vi "DHE_ParseBinning.vi"(8 "error in":errorcluster, 10 "binning":string) -> (0 "error out":errorcluster, 2 "ybining":i32, 3 "xbining":i32)   [LabVIEW 2016]
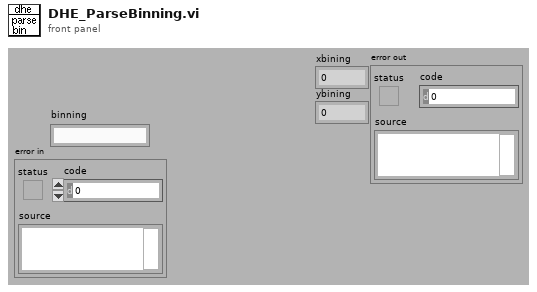
[diagram p1: front panel]
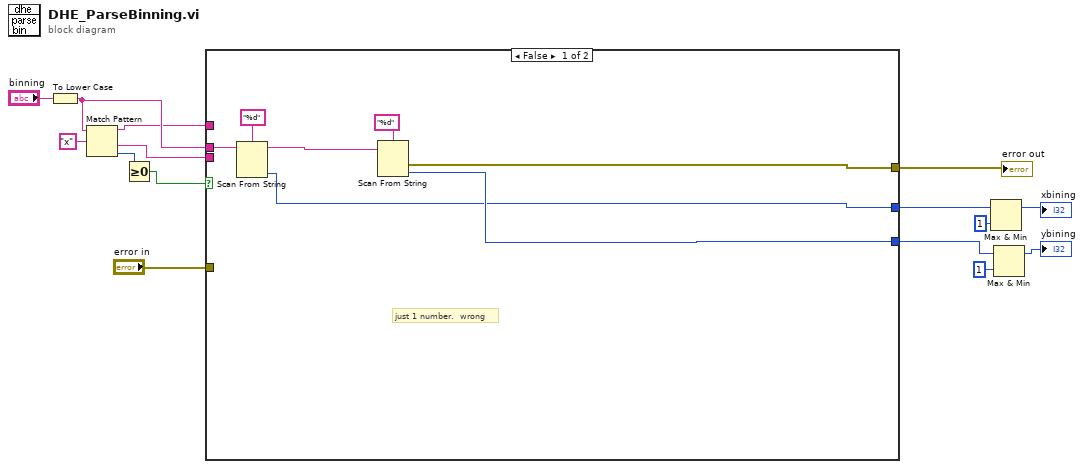
[diagram p0: block diagram]
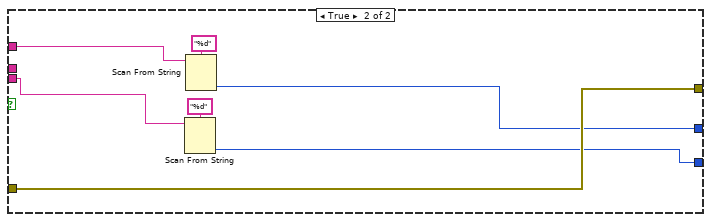
[diagram p2: hidden frame]
diagram:
  n1 = To Lower Case(string="binning") -> (all lower case string=w4:string)
  n2 = Match Pattern(string=w4, regular expression="x") -> (before substring=w2:string, after substring=w1:string, offset past match=w7:i32)  [unwired: 2 out]
  n3 = Greater Or Equal To 0?(x=w7) -> (x >= 0?=w3:bool)
  n4 = case shown="False" w3 {
    tunnel: [w20 w25] -> w15
    tunnel: "error in" -> [_ w25]
    tunnel: [w19 w23] -> w13
    tunnel: [w18 w24] -> w11
    tunnel: w4 -> [w17 _]
    tunnel: w2 -> [_ w27]
    tunnel: w1 -> [_ w26]
    frame False {
      # "just 1 number.  wrong"
      n5 = Scan From String(format string="%d", input string=w17) -> (remaining string=w21:string, output 1=w18:i32)  [unwired: 2 in, 3 out]
      n6 = Scan From String(format string="%d", input string=w21) -> (error out=w20:errorcluster, output 1=w19:i32)  [unwired: 2 in, 3 out]
    }
    frame True {
      n7 = Scan From String(format string="%d", input string=w26) -> (output 1=w23:i32)  [unwired: 2 in, 4 out]
      n8 = Scan From String(format string="%d", input string=w27) -> (output 1=w24:i32)  [unwired: 2 in, 4 out]
    }
  }
  "error out" <- w15
  n9 = Max & Min(x=w11, y=1) -> (max(x,y)=→"xbining":i32)  [unwired: 1 out]
  n10 = Max & Min(x=w13, y=1) -> (max(x,y)=→"ybining":i32)  [unwired: 1 out]
